vi "Get Primary Destination Path.vi"(8 "error in (no error)":errorcluster, 11 "PPL in":refnum<class "NI_AB_API_DPPL.lvclass">) -> (0 "error out":errorcluster, 2 "Primary destination path":path, 3 "PPL out":refnum<class "NI_AB_API_DPPL.lvclass">)   [LabVIEW 2020, in "NI_AB_API_DPPL.lvclass"]
uses:
  <vilib>/AppBuilder/AB_API/DPPL/NI_AB_API_DPPL.lvclass
  <vilib>/AppBuilder/AB_API/PPL/NI_AB_API_PPL.lvclass
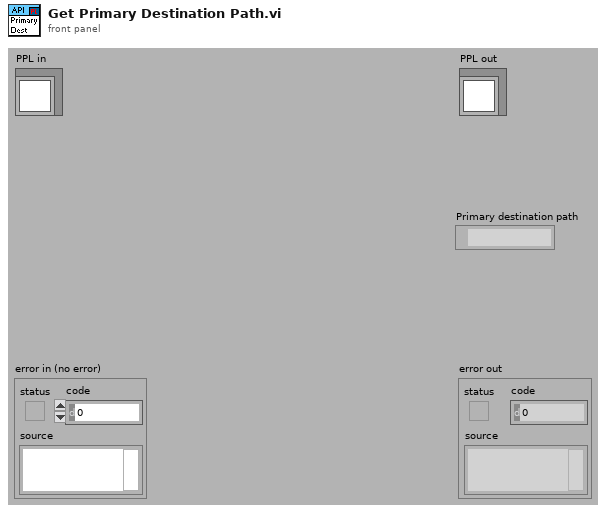
[diagram p1: front panel]
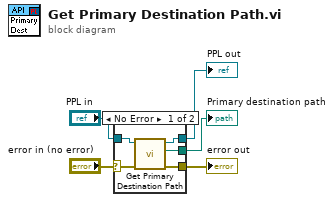
[diagram p0: block diagram]
diagram:
  n1 = case shown="No Error" "error in (no error)" {
    selector: "error in (no error)" -> [w7 w11]
    tunnel: [w6 w11] -> w4
    tunnel: [w9 w12] -> w2
    tunnel: "PPL in" -> [w10 w12]
    tunnel: [w8 _] -> w1
    frame No Error {
      n2 = call-parent "Get Primary Destination Path.vi"("error in (no error)"=w7, "PPL in"=w10) -> ("error out"=w6:errorcluster, "Primary destination path"=w8:path, "PPL out"=w9:refnum<class "NI_AB_API_DPPL.lvclass">)  [unwired: 7 in]
    }
    frame Error {
    }
  }
  "error out" <- w4
  "PPL out" <- w2
  "Primary destination path" <- w1
